vi "Write Cfg String.vi"(8 "error in (no error)":errorcluster, 10 "Cfg String":string, 11 "Get Serialized Device Configuration MSG in":refnum<class "Get Serialized Device Configuration MSG.lvclass">) -> (0 "error out":errorcluster, 3 "Get Serialized Device Configuration MSG out":refnum<class "Get Serialized Device Configuration MSG.lvclass">)   [LabVIEW 2014]
uses:
  Get Serialized Device Configuration MSG.lvclass
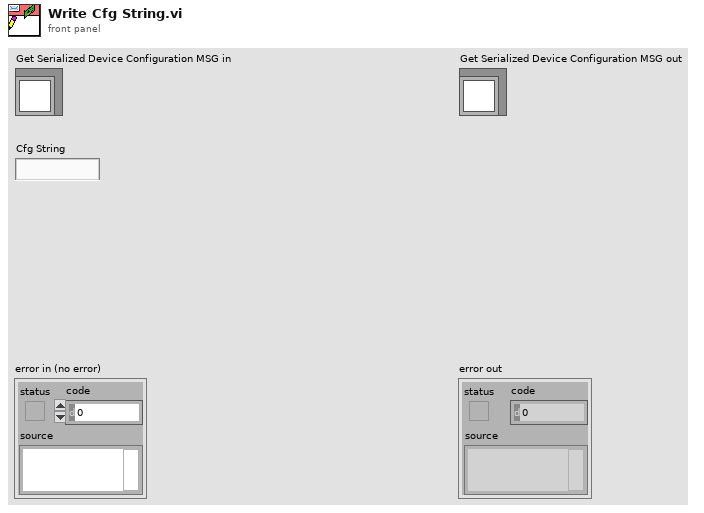
[diagram p1: front panel]
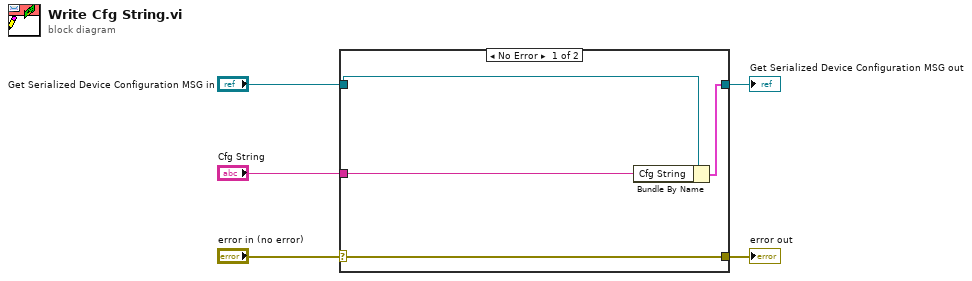
[diagram p0: block diagram]
diagram:
  n1 = case shown="No Error" "error in (no error)" {
    selector: "error in (no error)" -> [w9 w10]
    tunnel: [w9 w10] -> w4
    tunnel: [w7 w11] -> w2
    tunnel: "Get Serialized Device Configuration MSG in" -> [w8 w11]
    tunnel: "Cfg String" -> [w6 _]
    frame No Error {
      n2 = Bundle By Name(cluster=w8, "Cfg String"=w6) -> (w7:cluster{})
    }
    frame Error {
    }
  }
  "error out" <- w4
  "Get Serialized Device Configuration MSG out" <- w2
